vi "PV HLT5xx Operating turbopump.vi"(8 "error in (no error)":errorcluster, 9 "Operating adjustment - Cluster":T1={"Parameter"=0, "Parameter\nread only<->describe"=FALSE, "Motor Turbopump\noff<->on"=TRUE, "End of measuring\nrange of gauge"=0} {"End of measuring\nrange of gauge" items=[" 0,1 mbar", " 1 mbar", " 10 mbar", " 100 mbar", " 1000 mbar", " 2000 mbar", " 5000 mbar", " 10000 mbar", " 50000 mbar"]; "Parameter" items=[" End of measuring range of gauge", " Motor Turbopump", " Actual rotation speed TMP [Hz] (read only)", " Motor current TMP [A] (read only)", " Software version electronic drive unit  (read only)", " Operating hours TMP [h] (read only)", " Unit type electronic drive unit (read only)"]}, 10 "Adress of unit":u16=1 min=1 max=999 step=1, 11 "VISA session":refnum<visa-resource-name>) -> (0 "error out":errorcluster, 2 "response (data)":string, 3 "dup VISA session":refnum<visa-resource-name>)   [LabVIEW 2016, in "Pfeiffer Vacuum.lvlib"]
doc: "There are 7 parameters available, only one of which can be enabled at a time. \n\n0 - End of measuring range of gauge (default) Para 016\n1 - Motor Turbopump Para 023\n2 - Actual rotation speed TMP [Hz] (read only) Para 309\n3 - Motor current TMP [A] (read only) Para 310\n4 - Software version electronic drive unit (read only) Para 312\n5 - Operating hours TMP [h] (read only) Para 314\n6 - Unit type electronic drive unit (read only) Para 349\n\nNote: The 2 controls right of this one will set the appropriate values for the selected parameter. Any settings for an parameter that is not selected will be ignored. If a value is out of range, it will be changed to either the upper or the lower limit of the range."
uses:
  Pfeiffer Vacuum.lvlib
  PV HLT5xx Operating Turbopump - Cluster.ctl
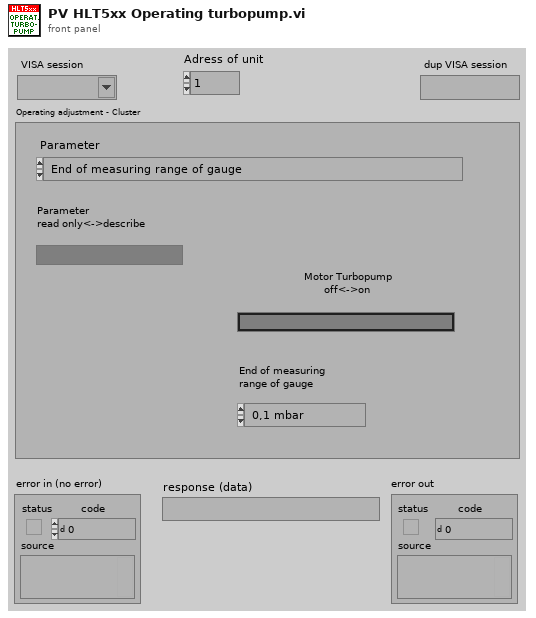
[diagram p1: front panel]
types:
  T1 = typedef "Pfeiffer Vacuum.lvlib/PV HLT5xx Operating Turbopump - Cluster.ctl" = cluster{"Parameter":u16, "Parameter\nread only<->describe":bool, "Motor Turbopump\noff<->on":bool, "End of measuring\nrange of gauge":u16}
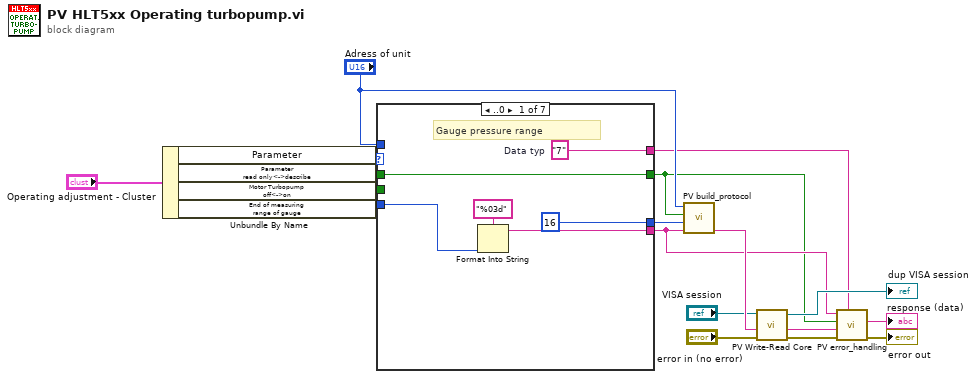
[diagram p0: block diagram]
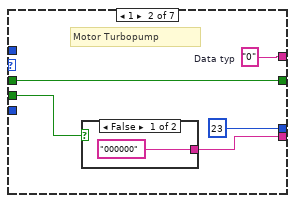
[diagram p2: hidden frame]
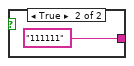
[diagram p3: hidden frame]
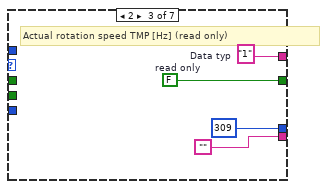
[diagram p4: hidden frame]
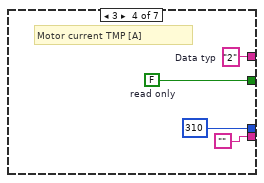
[diagram p5: hidden frame]
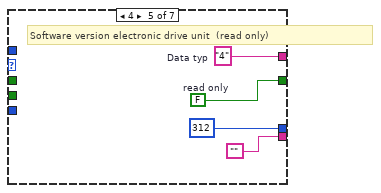
[diagram p6: hidden frame]
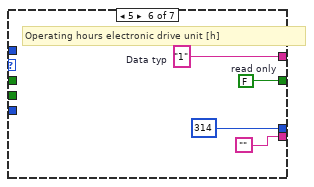
[diagram p7: hidden frame]
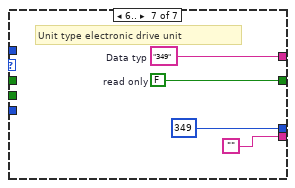
[diagram p8: hidden frame]
diagram:
  n1 = Unbundle By Name("Operating adjustment - Cluster") -> ("Parameter"=w1:u16, "Parameter\nread only<->describe"=w16:bool, "Motor Turbopump\noff<->on"=w15:bool, "End of measuring\nrange of gauge"=w2:u16)
  n2 = case shown="..0" w1 {
    tunnel: [u16 16 ("Parameter-number") u16 23 ("Parameter-number") u16 309 ("Parameter-number") u16 310 ("Parameter-number") u16 312 ("Parameter-number") u16 314 ("Parameter-number") u16 349 ("Parameter-number")] -> w18
    tunnel: [w20 w28 "" "" "" "" ""] -> w9
    tunnel: [w22 w27 w34 w38 w42 w44 w50] -> w7
    tunnel: w16 -> [w22 w27 _ _ _ _ _]
    tunnel: w15 -> [_ w26 _ _ _ _ _]
    tunnel: [w23 w25 w32 w39 w43 w47 w51] -> w8
    tunnel: "Adress of unit" -> [_ _ _ _ _ _ _]
    tunnel: w2 -> [w19 _ _ _ _ _ _]
    frame ..0 {
      w23 = "7"  # Data typ
      # "Gauge pressure range"
      n3 = Format Into String(format string="%03d" ("Format-String"), w19) -> (resulting string=w20:string)  [unwired: 2 in, 1 out]
    }
    frame 1 {
      w25 = "0"  # Data typ
      # "Motor Turbopump"
      n4 = case shown="False" w26 {
        tunnel: ["000000" ("Data") "111111" ("Data")] -> w28
        frame False {
        }
        frame True {
        }
      }
    }
    frame 2 {
      w32 = "1"  # Data typ
      w34 = FALSE  # read only
      # "Actual rotation speed TMP [Hz] (read only)"
    }
    frame 3 {
      w38 = FALSE  # read only
      w39 = "2"  # Data typ
      # "Motor current TMP [A]"
    }
    frame 4 {
      w43 = "4"  # Data typ
      w42 = FALSE  # read only
      # "Software version electronic drive unit  (read only)"
    }
    frame 5 {
      w44 = FALSE  # read only
      w47 = "1"  # Data typ
      # "Operating hours electronic drive unit [h]"
    }
    frame 6.. {
      w51 = "349"  # Data typ
      w50 = FALSE  # read only
      # "Unit type electronic drive unit"
    }
  }
  n5 = call "PV build_protocol.vi"("Data"=w9, "Parameter-number"=w18, "parameter\nread<->describe"=w7, "Adress"="Adress of unit") -> ("output"=w13:string)  [unwired: 3 in]
  n6 = call "PV Write-Read Core.vi"("error in"="error in (no error)", "Write data in"=w13, "VISA session"="VISA session") -> ("error out"=w11:errorcluster, "response (data) out"=w12:string, "dup VISA session"=→"dup VISA session":refnum<visa-resource-name>)  [unwired: 2 in]
  n7 = call "PV error_handling.vi"("Data Typ in"=w8, "error in"=w11, "response (data) in"=w12, "Parameter\nread only<->describe"=w7, "data in"=w9) -> ("error out"=→"error out":errorcluster, "Data out"=→"response (data)":string)  [unwired: 4 in, 1 out]
